vi "Write Header.vi"(8 "Error In":errorcluster, 9 "Current Time Stamp (now timestamp)":timestamp, 10 "Jig name (or acronym)":string, 11 "File refnum":refnum<file>) -> (0 "Error Out":errorcluster)   [LabVIEW 2023, in "Error Manager.lvlib" / "ErrorLog.lvlib"]
uses:
  ErrorLog.lvlib
panel:
  out "Text written to log":string
  # "Input\nInputs to the VI"
  # "Development\nControls or indicators that are useful for development or testing, but which are not outputs of the VI."
  # "Output\nOutputs of the VI"
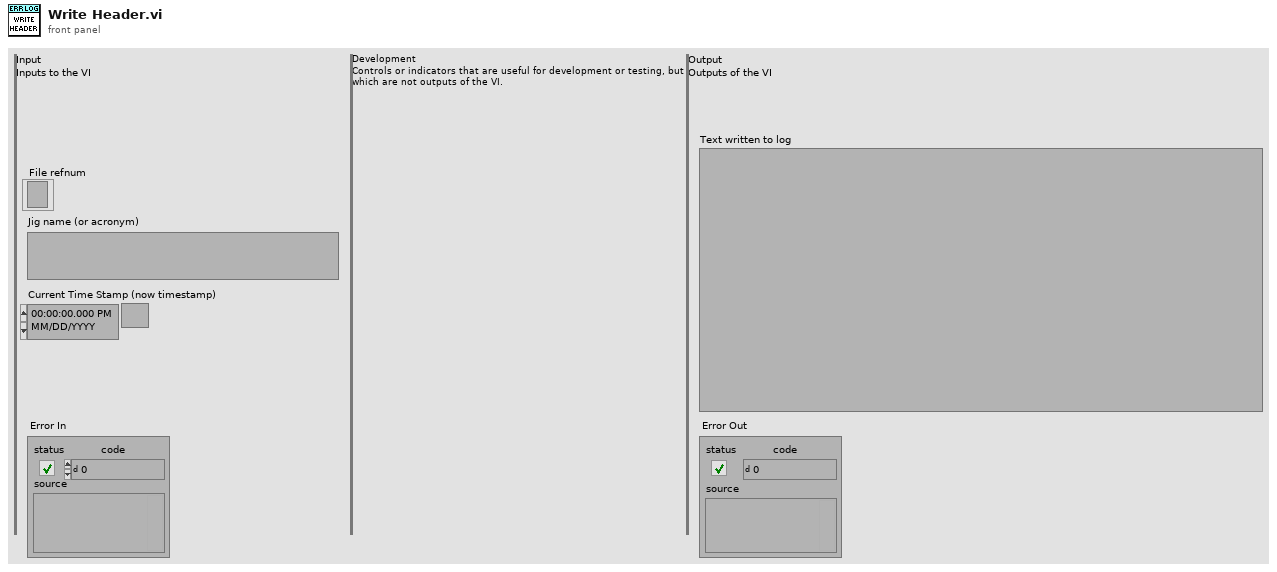
[diagram p1: front panel]
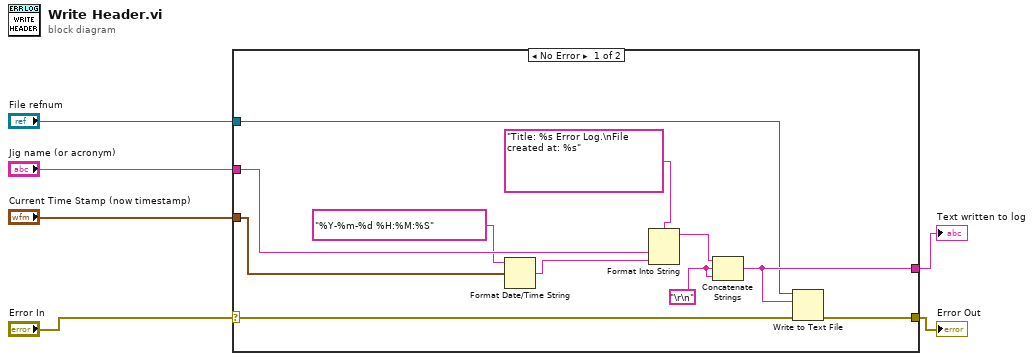
[diagram p0: block diagram]
diagram:
  n1 = case shown="No Error" "Error In" {
    selector: "Error In" -> [w16 w18]
    tunnel: [w17 w18] -> w5
    tunnel: "Current Time Stamp (now timestamp)" -> [w11 _]
    tunnel: "Jig name (or acronym)" -> [w12 _]
    tunnel: [w8 _] -> w2
    tunnel: "File refnum" -> [w7 _]
    frame No Error {
      w13 = "\r\n"
      n2 = Format Date/Time String(time format string (%c)="%Y-%m-%d %H:%M:%S", seconds (now)=w11) -> (date/time string=w9:string)  [unwired: 1 in]
      n3 = Format Into String(format string="Title: %s Error Log.\nFile created at: %s", w12, w9) -> (resulting string=w14:string)  [unwired: 2 in, 1 out]
      n4 = Concatenate Strings(w14, w13, w13) -> (w8:string)
      n5 = Write to Text File(file (use dialog)=w7, text=w8, error in=w16) -> (error out=w17:errorcluster)  [unwired: 1 in, 2 out]
    }
    frame Error {
    }
  }
  "Error Out" <- w5
  "Text written to log" <- w2
